vi "PH_SSAC.Save Data 2 Harddisk.vi"(1 "Instance Name":string, 2 "Date":string, 3 "Time":string, 4 "Time evolution of mean pulse duration [fs]":dbl[](array[numeric]), 5 "error in":errorcluster) -> (19 "error out":errorcluster)   [LabVIEW 2014, in "PH_SSAC.lvlib"]
uses:
  PH_SSAC.lvlib
  PH_Basics/PH_Common/Names/PH_Names.File Types.ctl
  PH_Basics/PH_Common/PH_Common.lvlib
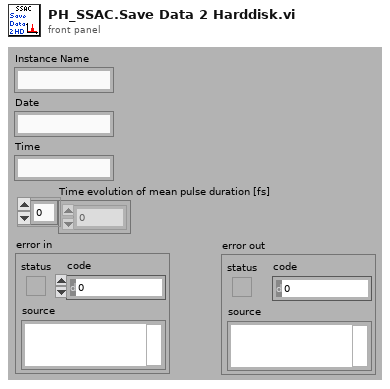
[diagram p1: front panel]
types:
  T1 = typedef "PH_Common.lvlib/PH_Names.File Types.ctl" = string
  T2 = enum16{"open", "replace", "create", "open or create", "replace or create", "replace or create with confirmation"}
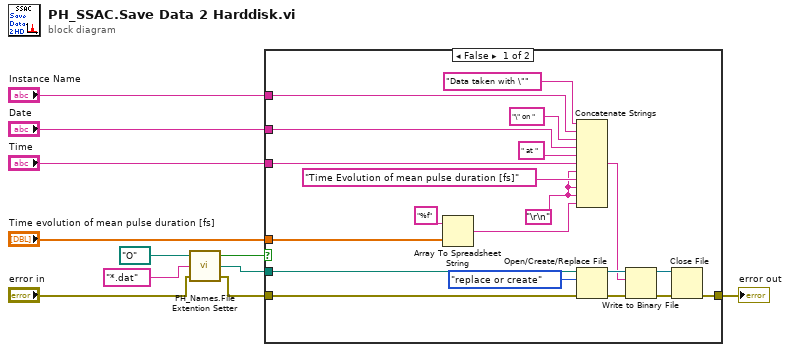
[diagram p0: block diagram]
diagram:
  n1 = call "PH_Names.File Extention Setter.vi"("error in (no error)"="error in", "File Type"=T1 "*.dat" ("file name extinction"), "start path (O:\\)"=path "O:/" ("start path (O:\\)")) -> ("error out"=w1:errorcluster, "path with extension"=w7:path, "cancelled?"=w3:bool)
  n2 = case shown="False" w3 {
    tunnel: "Instance Name" -> [w28 _]
    tunnel: "Date" -> [w26 _]
    tunnel: "Time" -> [w24 _]
    tunnel: [w22 w32] -> w8
    tunnel: w1 -> [w21 w32]
    tunnel: w7 -> [w20 _]
    tunnel: "Time evolution of mean pulse duration [fs]" -> [w13 _]
    frame False {
      w29 = "\r\n"
      n3 = Array To Spreadsheet String(array=w13, 3:"%f" ("format string")) -> (spreadsheet string=w23:string)  [unwired: 1 in]
      n4 = Concatenate Strings("Data taken with \"" ("string"), w28, "\" on " ("string"), w26, " at " ("string"), w24, w29, "Time Evolution of mean pulse duration [fs]" ("string"), w29, w29, w23) -> (w15:string)
      n5 = Open/Create/Replace File(file path (use dialog)=w20, error in=w21, operation (0:open)=T2."replace or create") -> (refnum out=w19:refnum<file>, error out=w17:errorcluster)  [unwired: 3 in, 1 out]
      n6 = Write to Binary File(file (use dialog)=w19, data=w15, error in=w17) -> (refnum out=w16:refnum<file>, error out=w18:errorcluster)  [unwired: 3 in, 1 out]
      n7 = Close File(refnum=w16, error in=w18) -> (error out=w22:errorcluster)  [unwired: 1 out]
    }
    frame True {
    }
  }
  "error out" <- w8
